vi "subXMLGetSourceItemInclusion.vi"(9 "index (1)":u32=1, 11 "Refnum in":refnum<k20>) -> (3 "Include?":bool)   [LabVIEW 2019, in "SolutionBuilder.lvlib" / "SolutionBuilder.lvclass"]
uses:
  SolutionBuilder.lvclass
  <vilib>/xml/NI_XML.lvlib
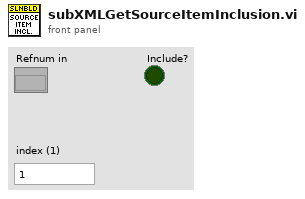
[diagram p1: front panel]
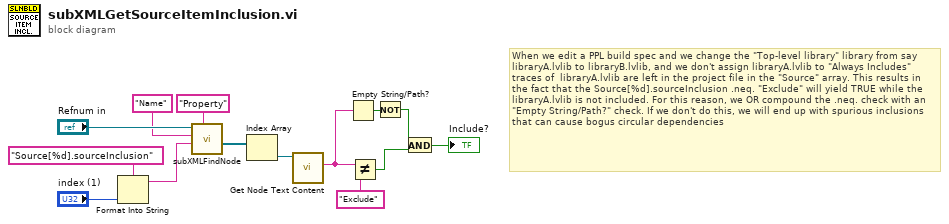
[diagram p0: block diagram]
diagram:
  # "When we edit a PPL build spec and we change the \"Top-level library\" library from say libraryA.lvlib to libraryB.lvlib, and we don't assign libraryA.lvlib to \"Always Includes\" traces of  libraryA.lvlib are left in the project file in the \"Source\" array. This results in the fact that the Source[%d].sourceInclusion .neq. \"Exclude\" will yield TRUE while the libraryA.lvlib is not included. For this reason, we OR compound the .neq. check with an \"Empty String/Path?\" check. If we don't do this, we will end up with spurious inclusions that can cause bogus circular dependencies"
  n1 = Format Into String(format string="Source[%d].sourceInclusion" ("Property value"), "index (1)") -> (resulting string=w8:string)  [unwired: 2 in, 1 out]
  n2 = call "subXMLFindNode.vi"("Node name"="Property", "Property value"=w8, "Property name"="Name", "Refnum in"="Refnum in") -> ("Nodes"=w12:refnum<k20>[])  [unwired: 6 in, 1 out]
  n3 = Index Array(array=w12) -> (element=w13:refnum<k20>)  [unwired: 1 in]
  n4 = call <vilib>:"Get Node Text Content.vi"("node in"=w13) -> ("node text"=w5:string)  [unwired: 8 in, 2 out]
  n5 = Empty String/Path?(string/path=w5) -> (empty?=w3:bool)
  n6 = Not Equal?(x=w5, y="Exclude" ("regular expression")) -> (x != y?=w4:bool)
  n7 = Not(x=w3) -> (.not. x?=w1:bool)
  n8 = And(x=w1, y=w4) -> (x .and. y?=→"Include?":bool)
